vi "Finish.vi"   [LabVIEW 2019]
doc: "This VI is called just before exiting. It is expected to close I/O refnum, save collected data, etc."
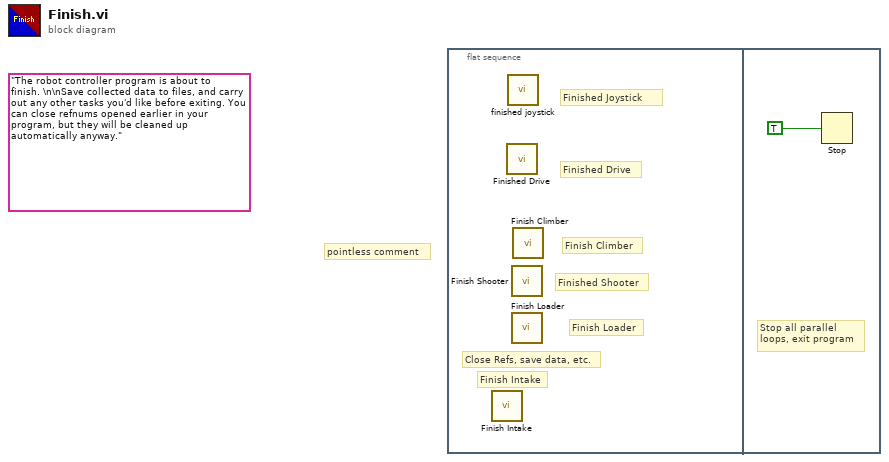
[diagram p0: block diagram]
diagram:
  (unwired) "The robot controller program is about to finish. \n\nSave collected data to files, and carry out any other tasks you'd like before exiting. You can close refnums opened earlier in your program, but they will be cleaned up automatically anyway."
  # "pointless comment"
  n1 = flat-sequence {
    frame #0 {
      # "Finish Climber"
      # "Finish Intake"
      # "Finish Loader"
      # "Finished Shooter"
      # "Finished Drive"
      # "Finished Joystick"
      # "Close Refs, save data, etc."
      n2 = call "Finish Intake.vi"() -> ()  [unwired: 12 in]
      n3 = call "Finished Drive.vi"() -> ()  [unwired: 12 in]
      n4 = call "finished joystick.vi"() -> ()  [unwired: 12 in]
      n5 = call "Finish Shooter.vi"() -> ()  [unwired: 12 in]
      n6 = call "Finish Loader.vi"() -> ()  [unwired: 12 in]
      n7 = call "Finish Climber.vi"() -> ()  [unwired: 12 in]
    }
    frame #1 {
      # "Stop all parallel\nloops, exit program"
      n8 = Stop(stop? (T)=TRUE ("Quit")) -> ()
    }
  }
